vi "Image Alignment.vi"(8 "smoothing radius":u16=1, 10 "Image 2":i16[][](graph), 11 "Image 1":i16[][](graph)) -> (0 "Rxy":dbl[][](graph) caption="Image 2", 1 "Y shift":i32, 3 "X shift":i32)   [LabVIEW 2018]
uses:
  <vilib>/Analysis/2dsp.llb/2D Cross Correlation (DBL).vi
  <vilib>/Analysis/NI_AALPro.lvlib
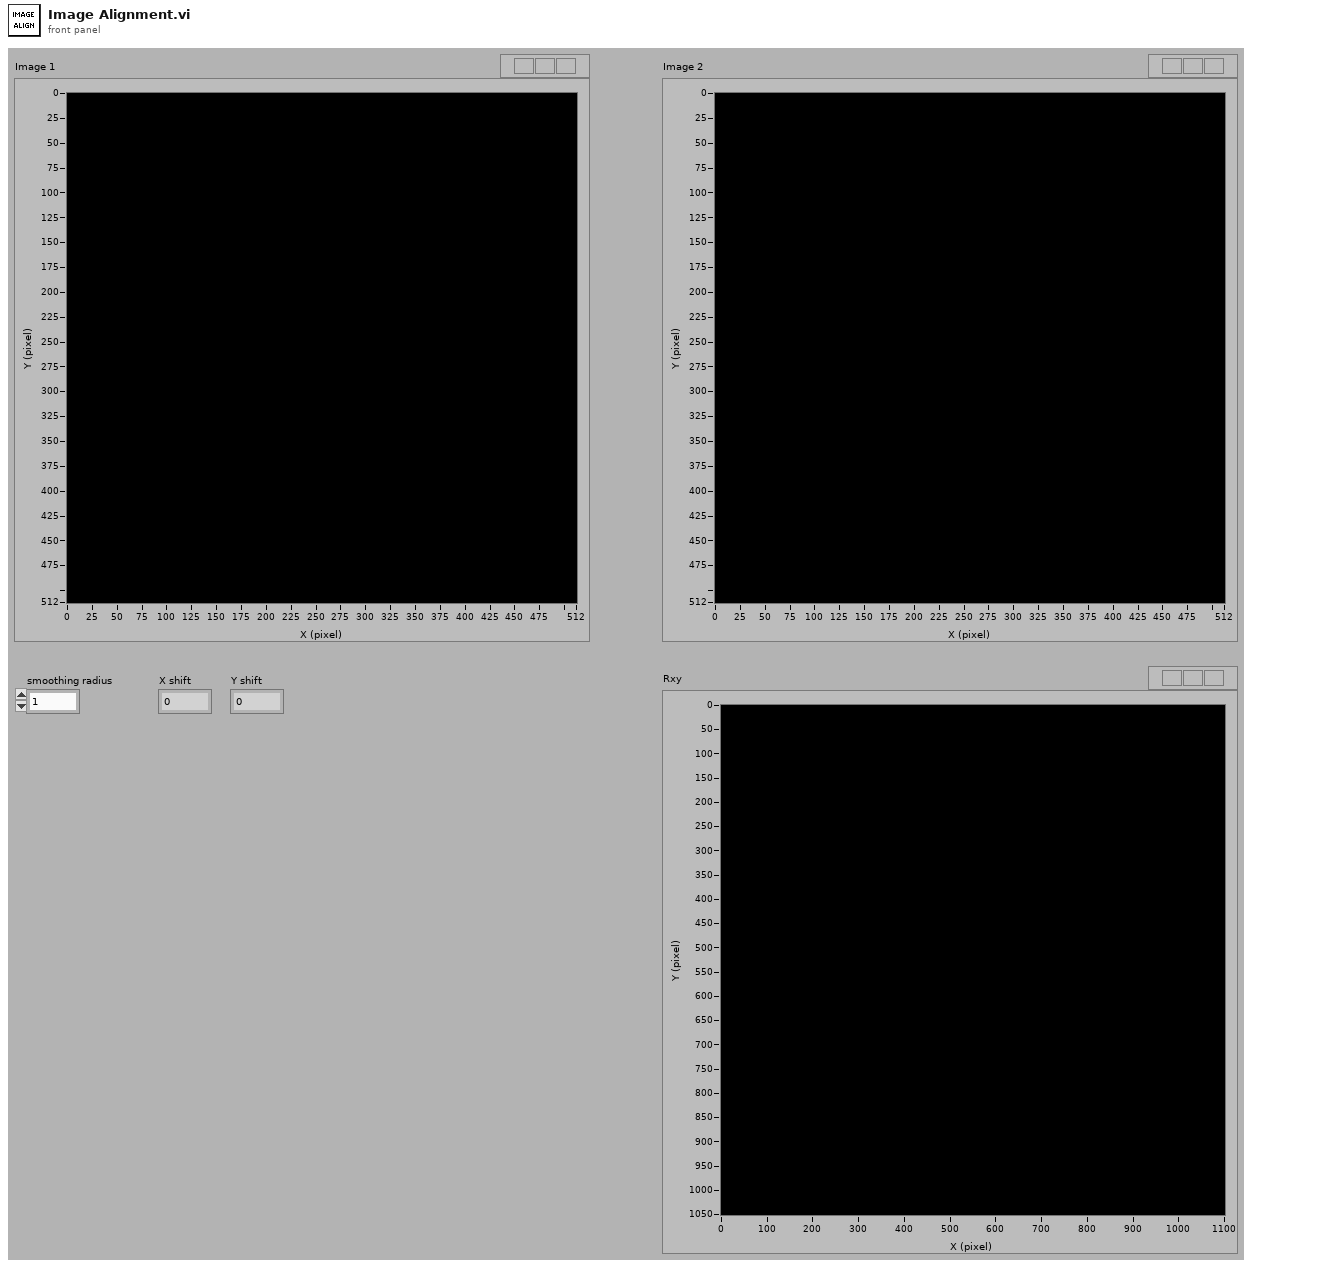
[diagram p1: front panel]
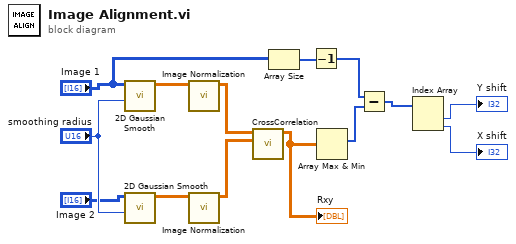
[diagram p0: block diagram]
diagram:
  n1 = call "2D Gaussian Smooth.vi"("radius"="smoothing radius", "Input"="Image 1") -> ("Output"=w4:dbl[][])  [unwired: 8 in, 1 out]
  n2 = call "2D Gaussian Smooth.vi"("radius"="smoothing radius", "Input"="Image 2") -> ("Output"=w2:dbl[][])  [unwired: 8 in, 1 out]
  n3 = call "Image Normalization.vi"("Input"=w4) -> ("Output"=w3:dbl[][])  [unwired: 10 in]
  n4 = call "Image Normalization.vi"("Input"=w2) -> ("Output"=w1:dbl[][])  [unwired: 10 in]
  n5 = call-poly <vilib>:"CrossCorrelation.vi"("Y"=w1, "X"=w3) -> ("Rxy"=w7:dbl[][])  [unwired: 8 in, 1 out]
  "Rxy" <- w7
  n6 = Array Size(array="Image 1") -> (size(s)=w13:i32[])
  n7 = Decrement(x=w13) -> (x-1=w12:i32[])
  n8 = Array Max & Min(array=w7) -> (max index (indices)=w11:i32[])  [unwired: 3 out]
  n9 = Subtract(x=w12, y=w11) -> (x-y=w10:i32[])
  n10 = Index Array(array=w10) -> (element #1=→"Y shift":i32, element #2=→"X shift":i32)  [unwired: 2 in]
